vi "Init.vi"(7 "I2C #":T1=-1, 8 "error in (no error)":errorcluster, 10 "Session In":refnum<class "Session.lvclass">) -> (0 "error out":errorcluster, 2 "Version":string, 3 "Grove 2 RGB LED Matrix Out":refnum<class "Grove 2 RGB LED Matrix.lvclass">)   [LabVIEW 2020, in "CTI-Peripheral.lvlib" / "Grove 2 RGB LED Matrix.lvclass"]
uses:
  Grove 2 RGB LED Matrix.lvclass
  CTI/Session/Session.lvclass
  CTI/I2C Number.ctl
  CTI/I2C Address.ctl
  CTI/I2C Connection/I2C Connection.lvclass/I2C Connection.ctl
  Grove 2 RGB LED Matrix.lvclass/Grove 2 RGB LED Matrix.ctl
  CTI/I2C Connection/I2C Connection.lvclass
  CTI/CTI.lvlib
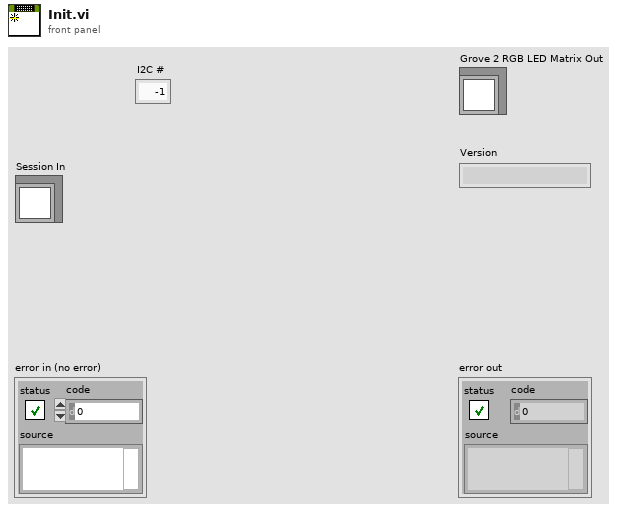
[diagram p1: front panel]
types:
  T1 = typedef "CTI.lvlib/I2C Number.ctl" = i8
  T2 = typedef "CTI.lvlib/I2C Address.ctl" = u8
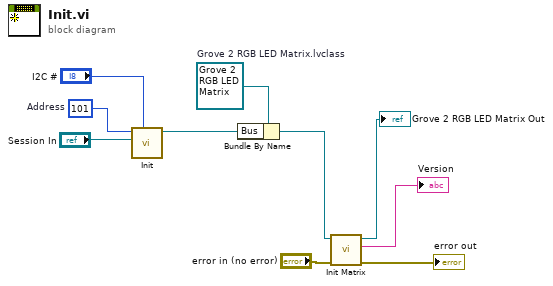
[diagram p0: block diagram]
diagram:
  w6 = refnum<class "Grove 2 RGB LED Matrix.lvclass"> refnum  # Grove 2 RGB LED Matrix.lvclass
  w7 = T2 101  # Address
  n1 = call "Init.vi"("I2C #"="I2C #", "Session"="Session In", "Address"=w7) -> ("I2C Connection"=w10:refnum<class "I2C Connection.lvclass">)  [unwired: 7 in, 1 out]
  n2 = Bundle By Name(cluster=w6, "Bus"=w10) -> (w5:refnum<class "Grove 2 RGB LED Matrix.lvclass">)
  n3 = call "Init Matrix.vi"("error in (no error)"="error in (no error)", "Grove 2 RGB LED Matrix in"=w5) -> ("error out"=→"error out":errorcluster, "Version"=→"Version":string, "Grove 2 RGB LED Matrix out"=→"Grove 2 RGB LED Matrix Out":refnum<class "Grove 2 RGB LED Matrix.lvclass">)  [unwired: 7 in]
